vi "subVI.vi"(11 "Variant":variant) -> (3 "Data Name":string)   [LabVIEW 2017]
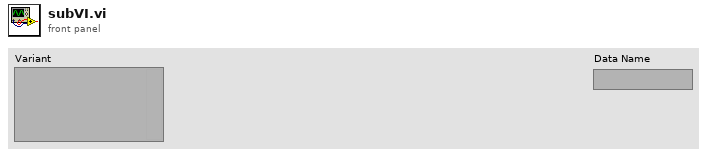
[diagram p1: front panel]
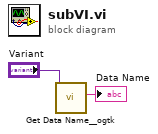
[diagram p0: block diagram]
diagram:
  n1 = call <userlib>:"Get Data Name__ogtk.vi"("Data"="Variant") -> ("Data Name"=→"Data Name":string)  [unwired: 8 in, 2 out]
